vi "TPosDSamp.vi"(0 "TPos Data":dbl[][](array[numeric]), 1 "Data Period (s)":dbl, 2 "TPos Disp. Dsamp":i32, 3 "Time Stamp":timestamp, 5 "Trap Pos":dbl[](array[numeric])) -> (14 "TPos dSampd":waveform(dbl)[](array[waveform]))   [LabVIEW 2013]
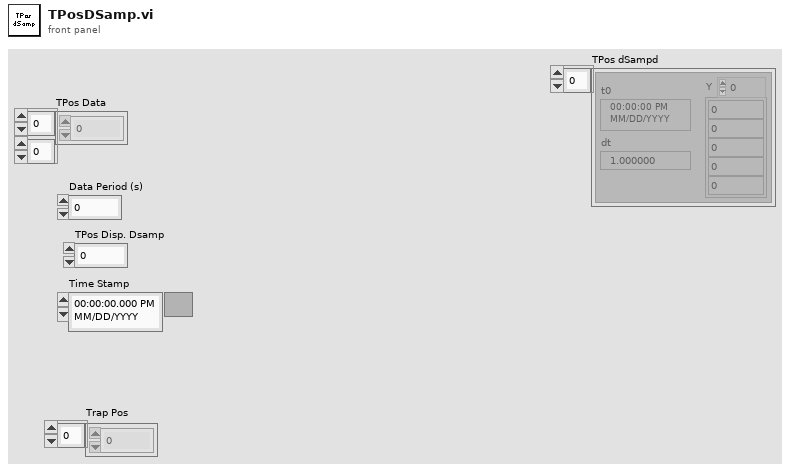
[diagram p1: front panel]
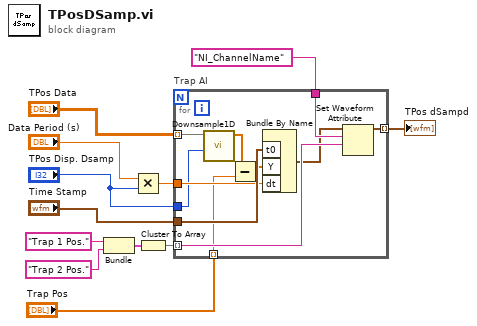
[diagram p0: block diagram]
diagram:
  n1 = Bundle("Trap 1 Pos.", "Trap 2 Pos.") -> (w2:cluster{string, string})  [unwired: 1 out]
  n2 = Multiply(x="Data Period (s)", y="TPos Disp. Dsamp") -> (x*y=w6:dbl)
  n3 = Cluster To Array(cluster=w2) -> (array=w1:string[])
  n4 = for "Trap AI" {
    tunnel: [w15] -> w9 mode=indexing
    tunnel: "Time Stamp" -> [w21]
    tunnel: "TPos Disp. Dsamp" -> [w18]
    tunnel: "TPos Data" -> [w19] mode=indexing
    tunnel: w1 -> [w23] mode=indexing
    tunnel: "NI_ChannelName" ("name") -> [w22]
    tunnel: w6 -> [w20]
    tunnel: "Trap Pos" -> [w13] mode=indexing
    n5 = call "Downsample1D.vi"("Avg N"=w18, "Array In"=w19) -> ("Array Out"=w17:dbl[])  [unwired: 9 in]
    n6 = Subtract(x=w17, y=w13) -> (x-y=w14:dbl[])
    n7 = Bundle By Name("t0"=w21, "Y"=w14, "dt"=w20) -> (w16:waveform(dbl))  [unwired: 1 out]
    n8 = Set Waveform Attribute(5:w23, 6:w22, 7:w16) -> (3:w15:waveform(dbl))  [unwired: 1 in, 2 out]
  }
  "TPos dSampd" <- w9
